vi "assembly_result_table_freq_char.vi"(8 "error_in":errorcluster, 9 "freq_values":dbl[](array[numeric])=[0.5, 2.0, 10.0, 20.0, 160.0, 2500.0, 4600.0, 4800.0] caption="Диапозон частот" min=0.0, 10 "measured_value":dbl[][](array[numeric]), 11 "RMS":dbl[][](array[numeric])) -> (0 "error_out":errorcluster, 3 "result_table_voltage":dbl[][](array[numeric]))   [LabVIEW 2017]
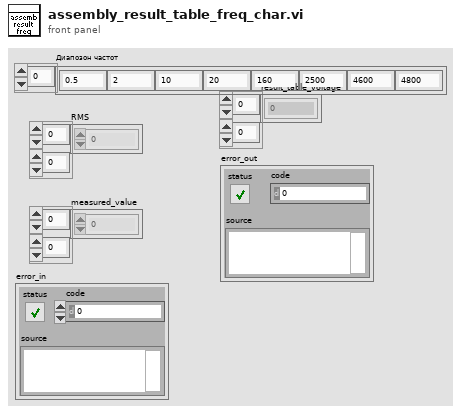
[diagram p1: front panel]
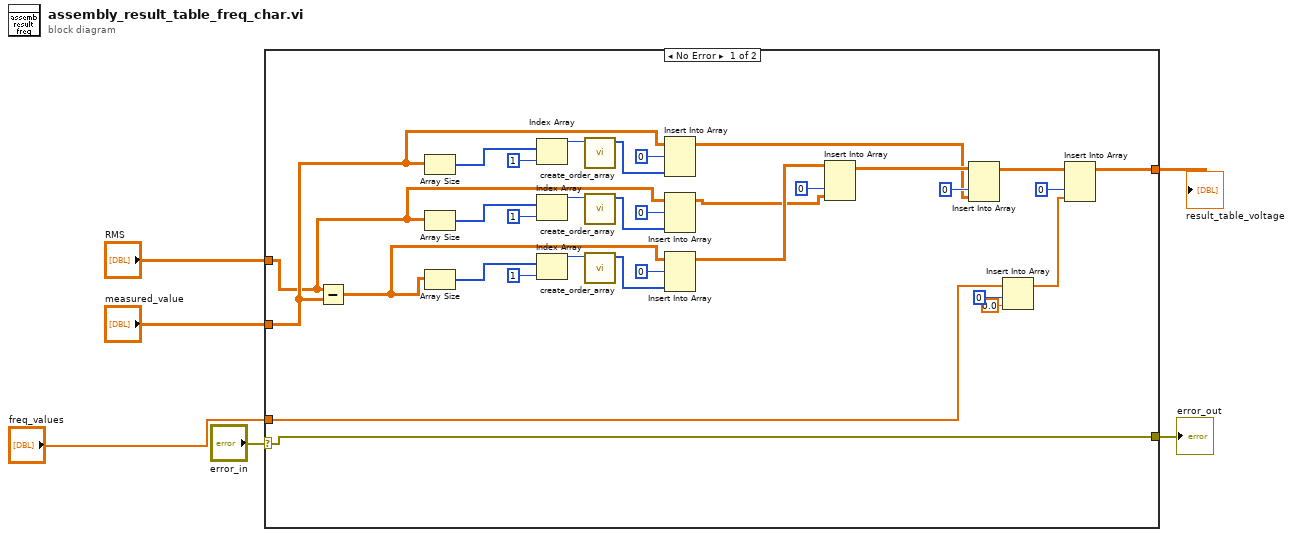
[diagram p0: block diagram]
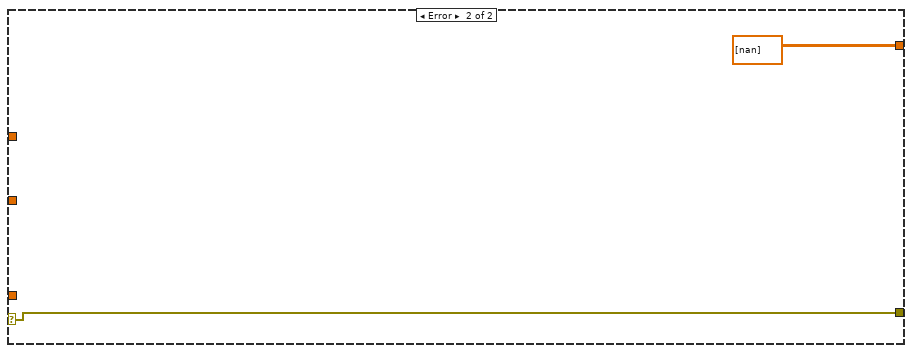
[diagram p2: hidden frame]
diagram:
  n1 = case shown="No Error" "error_in" {
    selector: "error_in" -> [w14 w40]
    tunnel: "measured_value" -> [w23 _]
    tunnel: "RMS" -> [w22 _]
    tunnel: [w11 dbl[][] [[nan]]] -> w4
    tunnel: [w14 w40] -> w3
    tunnel: "freq_values" -> [w10 _]
    frame No Error {
      n2 = Subtract(x=w22, y=w23) -> (x-y=w21:dbl[][])
      n3 = Array Size(array=w23) -> (size(s)=w37:i32[])
      n4 = Array Size(array=w22) -> (size(s)=w30:i32[])
      n5 = Array Size(array=w21) -> (size(s)=w27:i32[])
      n6 = Index Array(array=w37, index=1) -> (element=w36:i32)
      n7 = Index Array(array=w30, index=1) -> (element=w31:i32)
      n8 = Index Array(array=w27, index=1) -> (element=w26:i32)
      n9 = call "create_order_array.vi"("Numeric"=w36) -> ("Array"=w35:i32[])  [unwired: 10 in]
      n10 = call "create_order_array.vi"("Numeric"=w31) -> ("Array"=w32:i32[])  [unwired: 10 in]
      n11 = call "create_order_array.vi"("Numeric"=w26) -> ("Array"=w25:i32[])  [unwired: 10 in]
      n12 = Insert Into Array(array=w23, index (row)=0, new element=w35) -> (w15:dbl[][])  [unwired: 1 in]
      n13 = Insert Into Array(array=w22, index (row)=0, new element=w32) -> (w18:dbl[][])  [unwired: 1 in]
      n14 = Insert Into Array(array=w21, index (row)=0, new element=w25) -> (w20:dbl[][])  [unwired: 1 in]
      n15 = Insert Into Array(array=w20, index (col)=0 ("disabled index (col)"), new element=w18) -> (w16:dbl[][])  [unwired: 1 in]
      n16 = Insert Into Array(array=w16, index (col)=0 ("disabled index (col)"), new element=w15) -> (w13:dbl[][])  [unwired: 1 in]
      n17 = Insert Into Array(array=w10, index=0, new element=0.0 ("new element/subarray")) -> (w9:dbl[])
      n18 = Insert Into Array(array=w13, index (col)=0 ("disabled index (col)"), new element=w9) -> (w11:dbl[][])  [unwired: 1 in]
    }
    frame Error {
    }
  }
  "result_table_voltage" <- w4
  "error_out" <- w3
